vi "2 Message Logger.vi"() -> ()   [LabVIEW 2011]
uses:
  2 Classes/Logger/Logger.lvclass
panel:
  in  "Message Logger":refnum<class "Logger.lvclass">
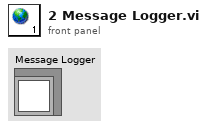
[diagram p1: front panel]
diagram:
